vi "Build Increment Numeric Functions.vi"   [LabVIEW 2021]
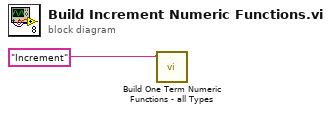
[diagram p0: block diagram]
diagram:
  n1 = call "Build One Term Numeric Functions - all Types.vi"("Comparison Name"="Increment") -> ()  [unwired: 11 in]
